vi "Toolbar Constant.vi"(10 "TBA Constant in":T2 {"Item"."Stop"."DisplayStyle" items=["None", "Text", "Image", "ImageAndText"]}) -> (2 "Toolbar":T2 {"Item"."Stop"."DisplayStyle" items=["None", "Text", "Image", "ImageAndText"]})   [LabVIEW 2016]
uses:
  SubVIs/TBA_NET_Item.ctl
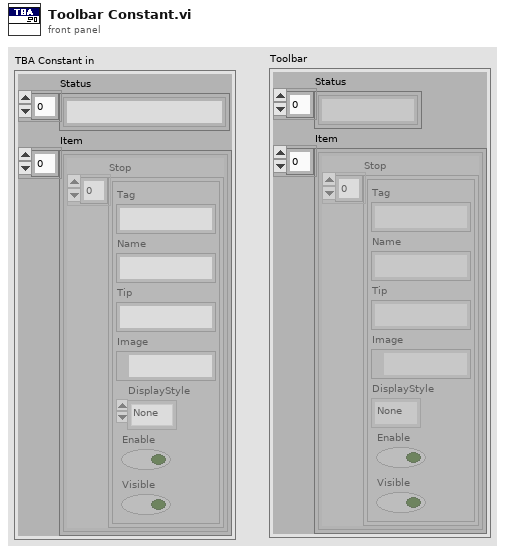
[diagram p1: front panel]
types:
  T1 = typedef "TBA_NET_Item.ctl" = cluster{"Tag":string, "Name":string, "Tip":string, "Image":path, "DisplayStyle":i32, "Enable":bool, "Visible":bool}
  T2 = cluster{"Status":string[], "Item":cluster{"Stop":T1[]}[]}
  T3 = enum32{"invalid app kind", "Development System", "Run Time System", "Student Edition", "Embedded LabVIEW", "Evaluation", "Custom"}
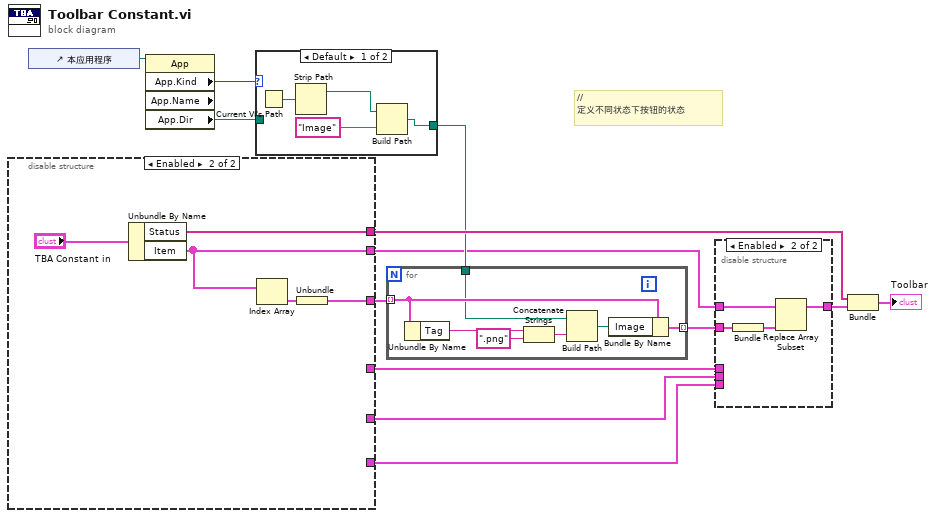
[diagram p0: block diagram]
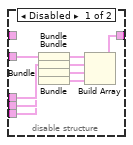
[diagram p2: hidden frame]
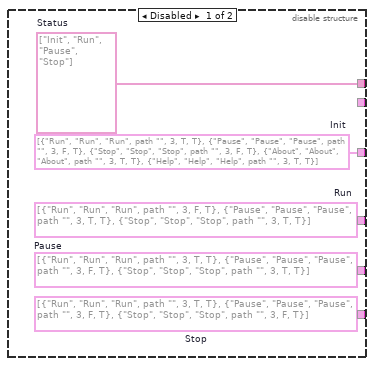
[diagram p3: hidden frame]
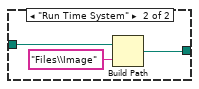
[diagram p4: hidden frame]
diagram:
  # "//\n定义不同状态下按钮的状态"
  n1 = disable-structure shown="Enabled" {
    disable-tunnel: [w18 w20] -> w13
    disable-tunnel: [w17 _] -> w11
    disable-tunnel: [w16 _] -> w10
    disable-tunnel: [w15 _] -> w9
    disable-tunnel: [w14 w22] -> w7
    disable-tunnel: [_ w19] -> w1
    frame Disabled {
      w14 = string[] ["Init", "Run", "Pause", "Stop"]  # Status
      w15 = T1[] [{"Tag"="Run", "Name"="Run", "Tip"="Run", "Image"=path "", "DisplayStyle"=3, "Enable"=TRUE, "Visible"=TRUE}, {"Tag"="Pause", "Name"="Pause", "Tip"="Pause", "Image"=path "", "DisplayStyle"=3, "Enable"=FALSE, "Visible"=TRUE}, {"Tag"="Stop", "Name"="Stop", "Tip"="Stop", "Image"=path "", "DisplayStyle"=3, "Enable"=FALSE, "Visible"=TRUE}]  # Stop
      w16 = T1[] [{"Tag"="Run", "Name"="Run", "Tip"="Run", "Image"=path "", "DisplayStyle"=3, "Enable"=TRUE, "Visible"=TRUE}, {"Tag"="Pause", "Name"="Pause", "Tip"="Pause", "Image"=path "", "DisplayStyle"=3, "Enable"=FALSE, "Visible"=TRUE}, {"Tag"="Stop", "Name"="Stop", "Tip"="Stop", "Image"=path "", "DisplayStyle"=3, "Enable"=TRUE, "Visible"=TRUE}]  # Pause
      w17 = T1[] [{"Tag"="Run", "Name"="Run", "Tip"="Run", "Image"=path "", "DisplayStyle"=3, "Enable"=FALSE, "Visible"=TRUE}, {"Tag"="Pause", "Name"="Pause", "Tip"="Pause", "Image"=path "", "DisplayStyle"=3, "Enable"=TRUE, "Visible"=TRUE}, {"Tag"="Stop", "Name"="Stop", "Tip"="Stop", "Image"=path "", "DisplayStyle"=3, "Enable"=TRUE, "Visible"=TRUE}]  # Run
      w18 = T1[] [{"Tag"="Run", "Name"="Run", "Tip"="Run", "Image"=path "", "DisplayStyle"=3, "Enable"=TRUE, "Visible"=TRUE}, {"Tag"="Pause", "Name"="Pause", "Tip"="Pause", "Image"=path "", "DisplayStyle"=3, "Enable"=FALSE, "Visible"=TRUE}, {"Tag"="Stop", "Name"="Stop", "Tip"="Stop", "Image"=path "", "DisplayStyle"=3, "Enable"=FALSE, "Visible"=TRUE}, {"Tag"="About", "Name"="About", "Tip"="About", "Image"=path "", "DisplayStyle"=3, "Enable"=TRUE, "Visible"=TRUE}, {"Tag"="Help", "Name"="Help", "Tip"="Help", "Image"=path "", "DisplayStyle"=3, "Enable"=TRUE, "Visible"=TRUE}]  # Init
    }
    frame Enabled {
      n2 = Unbundle By Name("TBA Constant in") -> ("Status"=w22:string[], "Item"=w19:cluster{"Stop":T1[]}[])
      n3 = Index Array(array=w19) -> (element=w21:cluster{"Stop":T1[]})  [unwired: 1 in]
      n4 = Unbundle(w21) -> ("Stop"=w20:T1[])
    }
  }
  n5 = control-ref of="本应用程序"() -> (w5:refnum<vi>)
  n6 = property class="App" props=["App.Kind", "App.Name", "App.Dir"](reference=w5) -> ("App.Kind"=w2:T3, "App.Dir"=w4:path)  [unwired: 1 in, 3 out]
  n7 = case shown="Default" w2 {
    tunnel: w4 -> [_ w30]
    tunnel: [w24 w29] -> w3
    frame Default {
      n8 = Current VI's Path() -> (path=w27:path)
      n9 = Strip Path(path=w27) -> (stripped path=w26:path)  [unwired: 1 out]
      n10 = Build Path(base path=w26, name or relative path="Image" ("名称或相对路径")) -> (appended path=w24:path)
    }
    frame "Run Time System" {
      n11 = Build Path(base path=w30, name or relative path="Files\\Image") -> (appended path=w29:path)
    }
  }
  n12 = for {
    tunnel: w13 -> [w37] mode=indexing
    tunnel: w3 -> [w36]
    tunnel: [w31] -> w12 mode=indexing
    n13 = Unbundle By Name(w37) -> ("Tag"=w35:string)
    n14 = Concatenate Strings(w35, ".png" ("字符串")) -> (w33:string)
    n15 = Build Path(base path=w36, name or relative path=w33) -> (appended path=w32:path)
    n16 = Bundle By Name(cluster=w37, "Image"=w32) -> (w31:T1)
  }
  n17 = disable-structure shown="Enabled" {
    disable-tunnel: w12 -> [w46 w47]
    disable-tunnel: w11 -> [w44 _]
    disable-tunnel: w10 -> [w43 _]
    disable-tunnel: w9 -> [w42 _]
    disable-tunnel: [w38 w49] -> w8
    disable-tunnel: w1 -> [_ w50]
    frame Disabled {
      n18 = Bundle(w46) -> (w45:cluster{T1[]})  [unwired: 1 in]
      n19 = Bundle("Run"=w44) -> (w41:cluster{"Run":T1[]})  [unwired: 1 in]
      n20 = Bundle("Pause"=w43) -> (w40:cluster{"Pause":T1[]})  [unwired: 1 in]
      n21 = Bundle("Stop"=w42) -> (w39:cluster{"Stop":T1[]})  [unwired: 1 in]
      n22 = Build Array(w45, w41, w40, w39) -> (w38:cluster{"Stop":T1[]}[])
    }
    frame Enabled {
      n23 = Bundle(w47) -> (w48:cluster{T1[]})  [unwired: 1 in]
      n24 = Replace Array Subset(array=w50, new element=w48) -> (w49:cluster{"Stop":T1[]}[])  [unwired: 1 in]
    }
  }
  n25 = Bundle("Status"=w7, "Item"=w8) -> (→"Toolbar":T2)  [unwired: 1 in]
